vi "Send Data.vi"() -> ()   [LabVIEW 2020, in "RT_Cluster.lvclass"]
uses:
  RT_Cluster.lvclass
  Desktop/efr_12/02_Electronics/VCU/Software/Project_EFR12e09/Typedefs/RT_Cluster.ctl
  Desktop/efr_12/02_Electronics/VCU/Software/Project_EFR12e09/Typedefs/RT_Vehicle_Modes.ctl
  RT_Cluster.lvclass/RT_Cluster.ctl
  <vilib>/Platform/TimedLoop/XDataNode/timing_clust.ctl
  <vilib>/Platform/TimedLoop/XDataNode/nitl_modes.ctl
  <vilib>/Platform/TimedLoop/XDataNode/wakeup.ctl
  944b02c2-96e3-4360-906f-94be907d6afc.vi
  52bb762b-3344-4100-a38b-be0fe8b4f671.vi
  743889c7-9139-4068-ac03-3bcab9db493b.vi
  7bc09824-a4a5-4f1b-b862-42a96e625018.vi
  c340d439-48fc-4ce6-b793-888df5355522.vi
  fd4fa075-0ab3-44ce-9a90-155efef00941.vi
  f70b0d1b-d714-4ea4-9e83-26cb66d79a99.vi
  c65facf9-95a3-4195-afb2-c6ea00a184ea.vi
  <vilib>/JDP Science/JSONtext/Variant to JSON Text.vi
  <vilib>/JDP Science/JSONtext/LVClass Serializer/JSONtext LVClass Serializer.lvclass
  <vilib>/platform/TimedLoop/XDataNode/XDataNode.xnode
  <vilib>/Platform/TimedLoop/XDataNode/XDNodeRunTimeDep.lvlib
panel:
  in  "Vehicle Mode":T1
  out "<JSON> 8":string
  out "<JSON> 7":string
  out "<JSON> 6":string
  out "<JSON> 5":string
  out "<JSON> 4":string
  out "<JSON> 3":string
  out "<JSON> 2":string
  out "<JSON>":string
  out "concatenated string":string
  out "xml string":string
  out "port":refnum<k16>
  out "send structure":dbl
  out "String 6":string
  out "Numeric":dbl
  out "String 5":string
  out "String 4":string
  out "String 2":string
  in  "stop 17":bool
  in  "stop 15":bool
  in  "stop 13":bool
  in  "stop 11":bool
  in  "stop 8":bool
  in  "stop 6":bool
  in  "stop 5":bool
  in  "stop 2":bool
  in  "Timestamp":cluster{"Timestamp":timestamp}
  in  "RT_Cluster.lvclass":T2
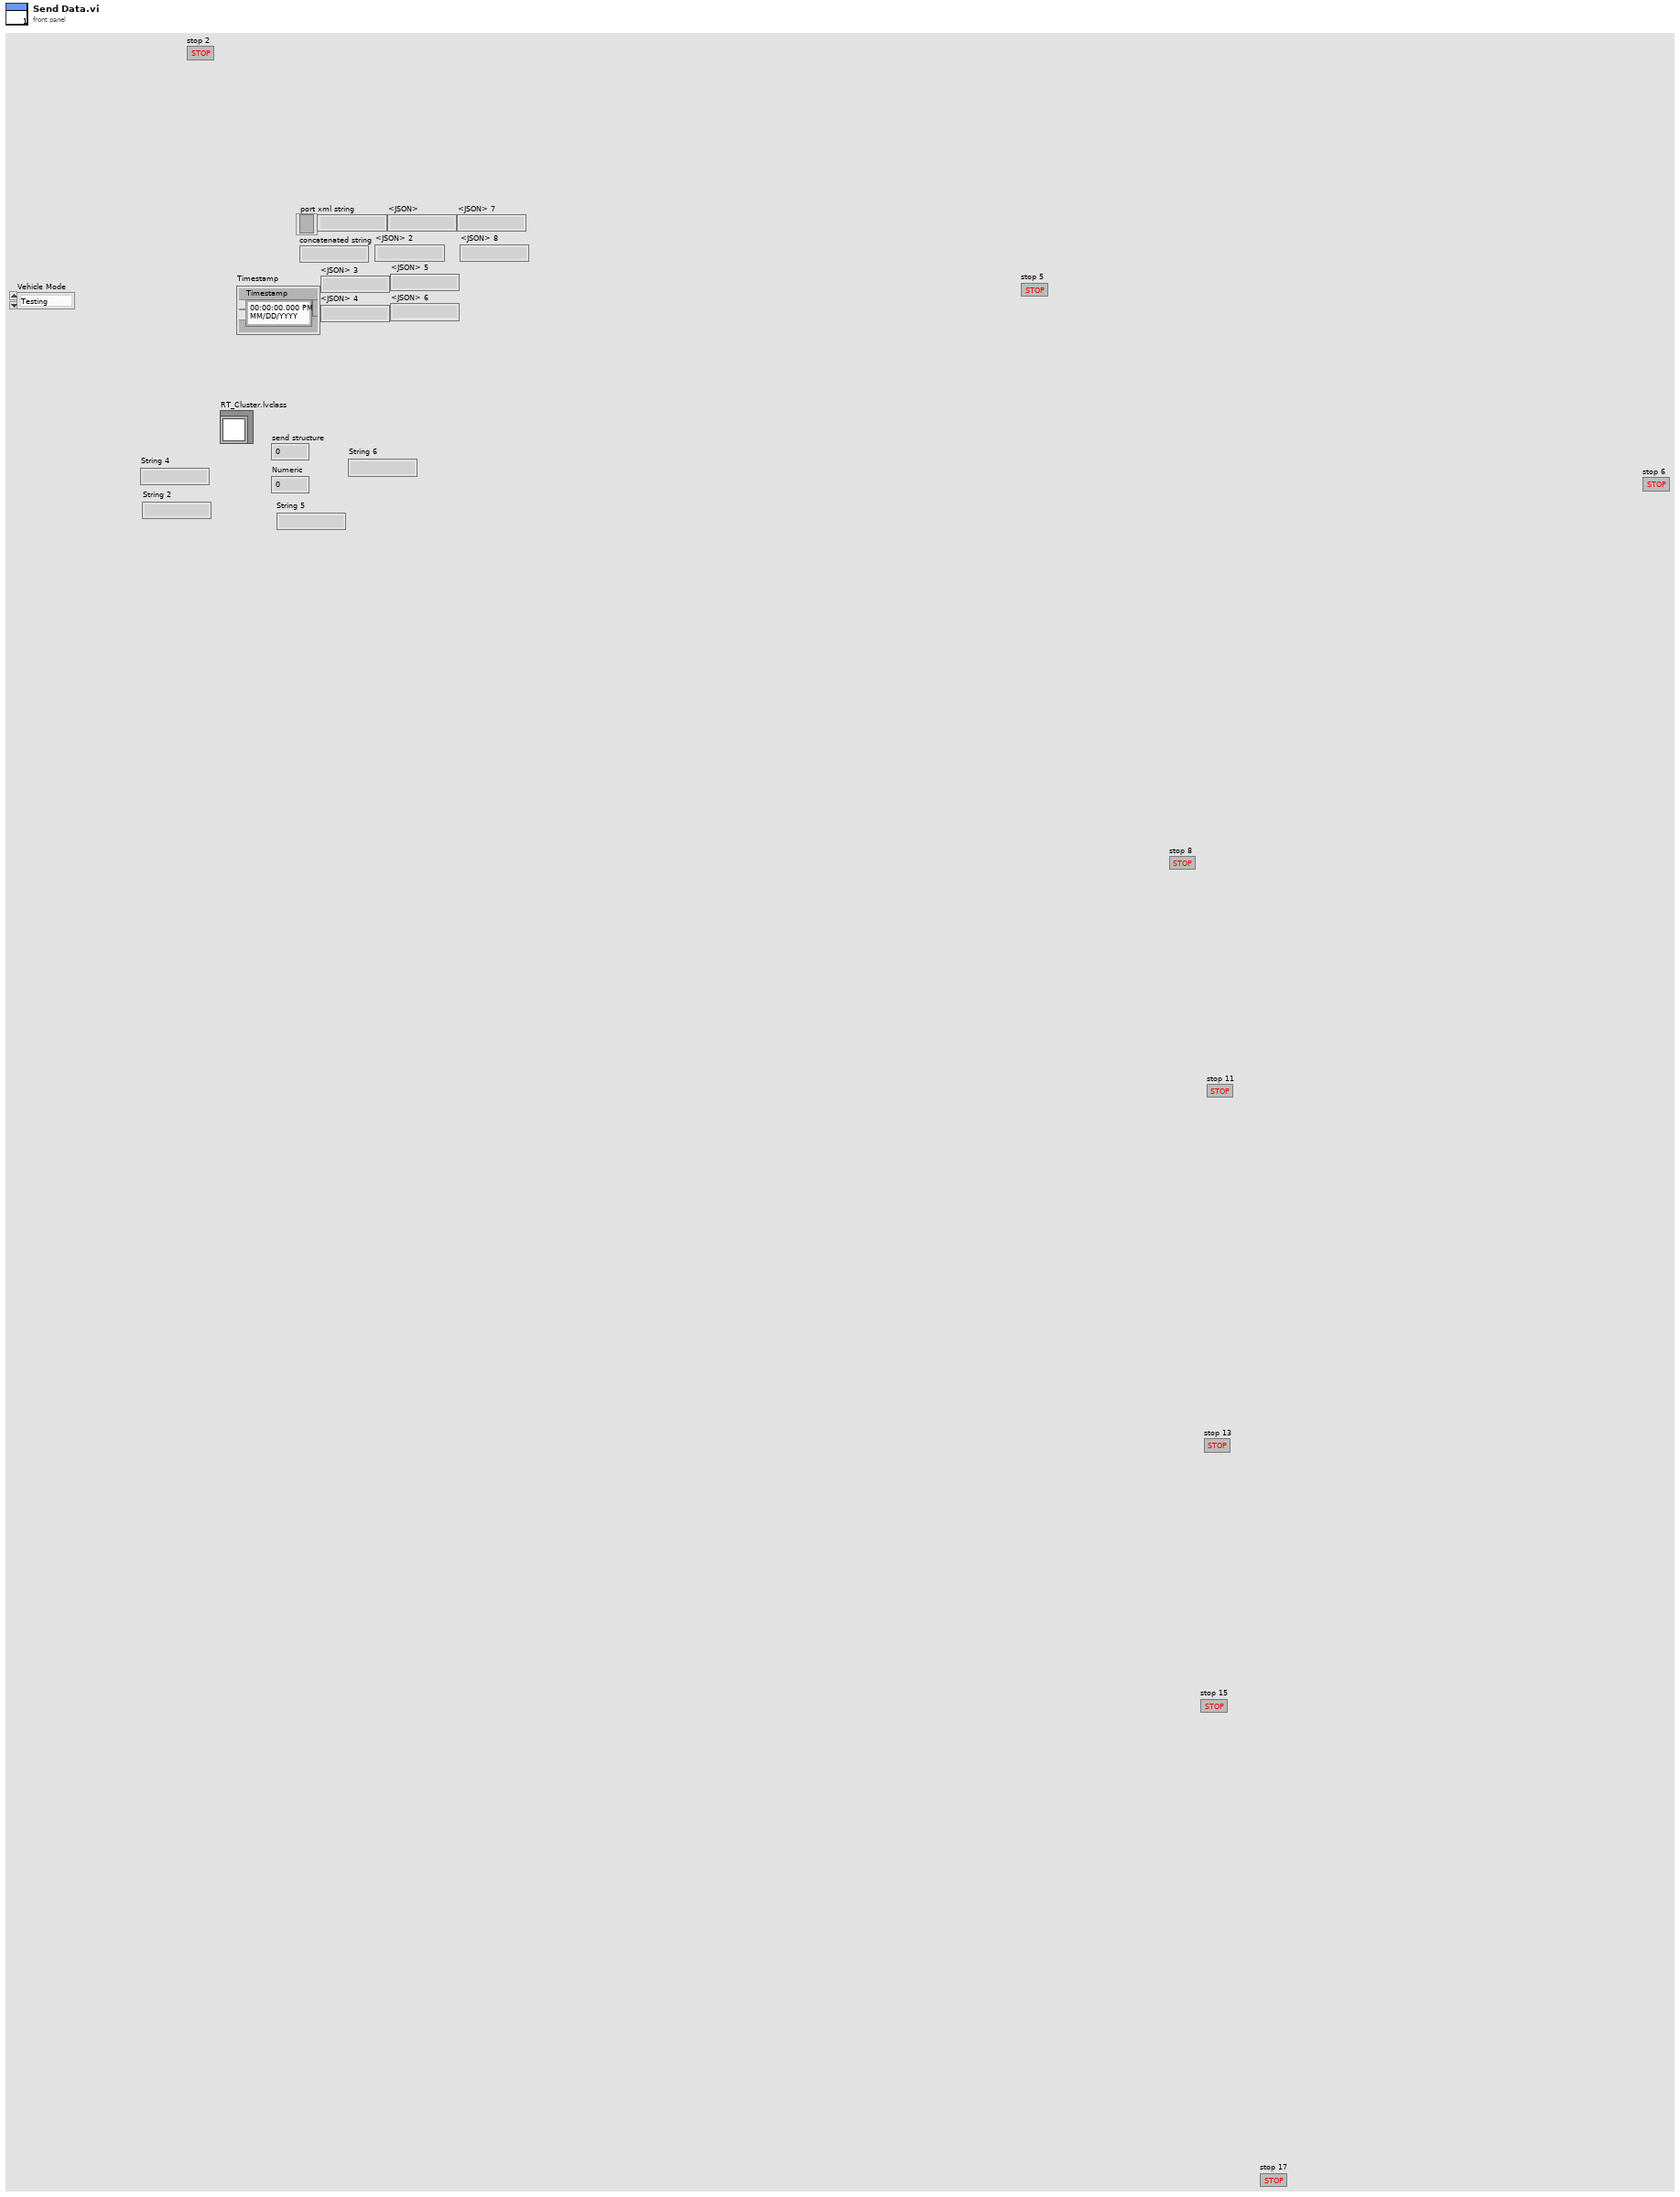
[diagram p1: front panel]
types:
  T1 = typedef "RT_Vehicle_Modes.ctl" = enum8{"Testing", "Scruti", "Acceleration", "Skidpad", "Autocross", "Endurance"}
  T2 = typedef "RT_Cluster.ctl" = refnum<class "RT_Cluster.lvclass">
  T3 = enum16{"big-endian, network order", "native, host order", "little-endian"}
  T4 = cluster{"Vehicle Mode":T1, "APPS1_min[°]":sgl, "APPS1_max[°]":sgl, "APPS2_min[°]":sgl, "APPS2_max[°]":sgl, "maxTorque+[Nm]":sgl, "maxTorque-[Nm]":sgl, "Leistungslimit[kW]":sgl, "maxRPM[1/min]":sgl, "Rekuperation":bool, "ASR":bool, "BSR":bool, "TV":bool, "DRS":bool, "Energiesparmodus":bool, "Accelslip [%/100]":sgl, "Brakeslip [%/100]":sgl, "Backupload":bool, "Config locked":bool, "InverterVR-active":bool, "InverterVL-active":bool, "InverterHR-active":bool, "InverterHL-active":bool}
  T5 = typedef "RT_AMS_States.ctl" = enum8{"Idle", "Precharging", "Drive", "reserved", "Precharge Failed", "Data Error", "Relay(s) stuck"}
  T6 = typedef "RT_IMD_States.ctl" = enum8{"IMD aus", "PWM nicht erkannt", "Normal", "Unterspannung", "Schnellstartmessung gut", "Schnellstartmessung schlecht", "Gerätefehler", "Anschlussfehler Erde"}
  T7 = typedef "FPGA_RT_Fuses.ctl" = cluster{"Fuse1[b]":bool, "Fuse2_SSB[b]":bool, "Fuse3_IMD[b]":bool, "Fuse4_Inv[b]":bool, "Fuse5_GPS[b]":bool, "Fuse6_VCU[b]":bool, "Fuse7_BSE[b]":bool, "Fuse8_DIS[b]":bool, "Fuse9_SWS[b]":bool, "Fuse10_TPMS[b]":bool, "Fuse11[b]":bool, "Fuse12[b]":bool, "Fuse1A_1_RTDS":bool, "Fuse1A_2_Brakelight":bool, "Fuse1A_3":bool, "Fuse1A_4":bool, "Fuse6A_1_Motor_Fans":bool, "Fuse6A_2_DRS":bool, "Fuse6A_3_SC":bool, "Fuse6A_4_Vectorbox":bool, "Fuse6A_5_Mot_Pumps":bool, "Fuse6A_6":bool, "Fuse12A_1_Inv_Fans_Fr":bool, "Fuse12A_2_Inv_Fans_Re":bool}
  T8 = cluster{"Analog":cluster{"APPS1[°]":sgl, "APPS2[°]":sgl, "Bremsdruck vorne [bar]":sgl, "Bremsdruck hinten [bar]":sgl, "Bremskraft[N]":sgl, "Lenkwinkel[°]":sgl, "WT_Motor_high[°C]":sgl, "WT_Motor_Low[°C]":sgl, "LT_Inv_FrR[°C]":sgl, "LT_Inv_FrL[°C]":sgl, "LT_Inv_ReR[°C]":sgl, "LT_Inv_ReL[°C]":sgl, "Ambient_Temp[°C]":sgl, "ST_FR[mm}":sgl, "ST_FL[mm]":sgl, "ST_RR[mm]":sgl, "ST_RL[mm]":sgl, "Temp_Fusebox [°C]":sgl}, "Akku/HV":cluster{"HV_Current[A]":sgl, "IC_Voltage[V]":sgl, "Charge[Ah]":sgl, "AMS-State":T5, "State SC":bool, "Akku-Voltage[V]":sgl, "SOC[%]":sgl, "CVH[V]":sgl, "CVL[V]":sgl, "CVL[V] 20s":sgl, "CVL[V] 60s":sgl, "CTH[°C]":sgl, "CTL[°C]":sgl, "State IMD":T6, "Isolationswider\nstand[kOhm]":u16}, "SC":cluster{"SC Messungen":cluster{"SC after Motors Rear [V]":sgl, "SC after Motors Front [V]":sgl, "SC after BOTS [V]":sgl, "SC after Akku [V]":sgl, "SC Voltage AMS 1":sgl, "SC Voltage AMS 2":sgl}, "SC Errors":cluster{"SC Motors Front":bool, "SC Motors Rear":bool, "SC BOTS":bool, "SC Akku":bool}}, "Fuses":T7, "Buttons/Knobs":cluster{"TunKnob 1[%]":sgl, "TunKnob 2[%]":sgl, "Start-Button":bool, "HV-Button":bool, "Reku-Button":bool, "Lenkrad 1":bool, "Lenkrad 2":bool, "Lenkrad 3":bool, "Lenkrad 4":bool, "Lenkrad 5":bool, "Lenkrad 6":bool}, "GPS/9-axis Front":cluster{"V_GPS[km/h]":sgl, "Course_GPS[°]":sgl, "Latitude[°]":dbl, "Longitude[°]":dbl, "HDOP":u8, "Quality of Fix":u8, "Satellites":u8, "Odometer[km]":sgl, "ACC_X_Fr[m/s²]":sgl, "ACC_Y_Fr[m/s²] ":sgl, "ACC_Z_Fr[m/s²]":sgl, "ROT_X_Fr[°/s]":sgl, "ROT_Y_Fr[°/s]":sgl, "ROT_Z_Fr[°/s]":sgl, "MAG_X_Fr[b]":sgl, "MAG_Y_Fr[b]":sgl, "MAG_Z_Fr[b]":sgl}, "GPS/9-axis Rear":cluster{"V_GPS[km/h]":sgl, "Course_GPS[°]":sgl, "Latitude[°]":dbl, "Longitude[°]":dbl, "HDOP":u16, "Quality of Fix":u16, "Satellites":u16, "Odometer[km]":sgl, "ACC_X_Re[m/s²]":sgl, "ACC_Y_Re[m/s²] ":sgl, "ACC_Z_Re[m/s²]":sgl, "ROT_X_Re[°/s]":sgl, "ROT_Y_Re[°/s]":sgl, "ROT_Z_Re[°/s]":sgl, "MAG_X_Re[b]":sgl, "MAG_Y_Re[b]":sgl, "MAG_Z_Re[b]":sgl}, "Fusebox Currents":cluster{"1A_1":sgl, "1A_ 2":sgl, "1A_3":sgl, "1A_4":sgl, "6A_1":sgl, "6A_2":sgl, "6A_3":sgl, "6A_4":sgl, "6A_5":sgl, "6A_6":sgl, "12A_1":sgl, "12A_2":sgl}, "Kistler":cluster{"Timestamp [4ms] ":u16, "IVI [10^-2 m/s]":u16, "Weg [m]":sgl, "V_lon [m/s]":sgl, "V_lat [m/s]":sgl, "Winkel [°]":sgl, "SerienNr":u32, "SensorNr":u8, "Temp [°C]":i8, "LED Strom [0,01A]":u8, "Statusbyte1":u8, "Statusbyte2":u8}, "Datalogger":cluster{"Status":u8, "Voltage[V]":sgl, "Current[A]":sgl, "Power[kW]":sgl, "Message\nCounter":sgl}}
  T9 = typedef "RT_Inverter.ctl" = cluster{"AMK_Control[b]":T10, "Drehzahlsollwert[1/min]":sgl, "Momentsollwert[Nm]":sgl, "System bereit":bool, "Warnung":bool, "Fehler":bool, "Derating":bool, "Spiegel HV":bool, "Quit HV":bool, "Spiegel Regelerfeigabe":bool, "Quit Reglerfreigabe":bool, "Drehzahlistwert[U/min]":sgl, "Momentistwert[Nm]":sgl, "Diagnosenummer":u16, "Motortemp[°C]":sgl, "Kühlplattentemp[°C]":sgl, "IGBTtemp[°C]":sgl, "I_q[A]":sgl, "I_d[A]":sgl, "Wirkleistung [kW]":sgl, "Blindleistung [kvar]":sgl, "Fehlerzusatznr. 1":u8, "Fehlerzusatznr. 2":u8, "Fehlerzusatznr. 3":u8}
  T10 = typedef "RT_AMK_Control.ctl" = enum8{"Fehler zurücksetzen", "HV-Freigabe", "HV+Antriebsfreigabe", "HV+Antriebs+Reglerfreigabe"}
  T11 = typedef "RT_Errors.ctl" = cluster{"Timeout CAN":T12, "Wert":cluster{"Pedale implausibel":bool, "APPS implausibel":bool, "APPS1":bool, "APPS2":bool, "Bremsdruck_vorne":bool, "Bremsdruck_hinten":bool, "Bremskraftsensor":bool, "Lenkwinkel":bool, "ACC_X":bool, "ACC_Y":bool, "ROT_Z":bool, "V_GPS":bool, "Invertertemp_FrR":bool, "Invertertemp_FrL":bool, "Invertertemp_ReR":bool, "Invertertemp_ReL":bool}, "Latching":cluster{"Pedale implausibel":bool, "APPS implausibel":bool, "APPS1":bool, "APPS2":bool}}
  T12 = typedef "FPGA_To_RT_CANErrors.ctl" = cluster{"SSB Front":bool, "BSE":bool, "SSB Rear":bool, "GPS Front":bool, "9-Achs_ACC Front":bool, "9-Achs_ROT Front":bool, "9-Achs_MAG Front":bool, "GPS Rear":bool, "9-Achs_ACC Rear":bool, "9-Achs_ROT Rear":bool, "9-Achs_MAG Rear":bool, "AMS":bool, "Energymeter":bool, "PDU":bool, "DIS":bool, "DIS_Param":bool, "Inverter FR":bool, "Inverter FL":bool, "Inverter RR":bool, "Inverter RL":bool}
  T13 = typedef "RT_Maths.ctl" = cluster{"General":cluster{"desiredTorque[Nm]":sgl, "Gaspedal[%/100]":sgl, "Rekupedal[%/100]":sgl, "Implausibilität\nAPPS[%]":sgl, "Bremsbal[Fr/Total]":sgl, "Accelbal[Fr/Total]":sgl, "allowedPower[kW]":sgl, "actualPower[kW]":sgl, "Energiesparmodus":bool, "Odometer":sgl, "Wirkungsgrad[%/100]":sgl, "T_Control[us]":sgl}, "TV/KF":cluster{"KF_Velocity[km/h]":sgl, "KF_ACC_X[m/s²]":sgl, "KF_slip_ist_FR[%/100]":sgl, "KF_slip_ist_FL[%/100]":sgl, "KF_slip_ist_RR[%/100]":sgl, "KF_slip_ist_RL[%/100]":sgl, "slip_soll_Fr[%/100]":sgl, "slip_soll_Re[%/100]":sgl, "TV_Regler[Giermoment]":sgl, "TV_Lenk[Giermoment]":sgl, "SOC-Soll[%]":sgl, "SOC-Ist[%]":sgl, "MomentSollVR[Nm]":sgl, "MomentSollVL[Nm]":sgl, "MomentSollHR[Nm]":sgl, "MomentSollHL[Nm]":sgl, "Reglerausgang":sgl}, "Energy Control":cluster{"allowedPower[kW]":sgl, "Rundenanzahl":sgl, "SOC-Soll[%]":sgl, "SOC-Ist[%]":sgl, "Rundenlänge[m]":sgl, "Reglerausgang":sgl, "Toleranz Rundenlänge [%/100]":sgl, "Strecke":T14, "Start-SOC[%]":sgl, "Ziel-SOC[%]":sgl, "Energie Akku[kWh]":sgl, "Maximalleistung[kW]":sgl, "Start-Leistungsgrenze":sgl}}
  T14 = typedef "RT_Tracks.ctl" = enum16{"Freital", "Barcelona", "Hockenheim", "Spielberg", "Assen"}
  T15 = typedef "RT_Vehicle_States.ctl" = enum8{"Idle", "Drive", "Error"}
  T16 = cluster{"Switches":cluster{"\n1A 1 RTDS":bool, "1A 2 Brakelight":bool, "1A 3":bool, "1A 4":bool, "6A 1 Motor Fans":bool, "6A 2 DRS":bool, "6A 3 SC":bool, "6A 4 Vectorbox":bool, "6A 5 Motor Pump":bool, "6A 6":bool, "12A 1 Inv Fans Fr":bool, "12A 2 Inv Fans Re":bool}, "Vehicle State":T15, "DRS Position[%/100]":sgl, "Fan Motor[%/100]":sgl, "Fan Akku[%/100]":sgl, "HV Freigabe ":bool, "IC Voltage OK":bool}
  T17 = cluster{"Input Error Code":i32, "Output Error Code":i32, "Transmit Error Counter":u8, " Error Counter":u32}
  T18 = typedef "XDNodeRunTimeDep.lvlib/timing_clust.ctl" = cluster{"Expected End [f-1]":u64, "Actual End [f-1]":u64, "Finished Late? [f-1]":bool, "Expected End [i-1]":u64, "Actual End [i-1]":u64, "Finished Late? [i-1]":bool, "Expected Start [i]":u64, "Actual Start [i]":u64, "Expected Start [f]":u64, "Actual Start [f]":u64, "Source Name":string, "Structure Name":string, "Period":i64, "Deadline":i64, "Offset":i64, "Start":i64, "Priority":i32, "Timeout":i32, "Mode":T19, "Wakeup Reason":T20, "Error":errorcluster, "Source Type":string, "Secondary Source Type":string, "Global End Time":u64, "Global Start Time":u64, "Frame Duration":u64, "Iteration Duration":u64, "Assigned CPU":i32, "I/O Scan Engine Mode":u32}
  T19 = typedef "XDNodeRunTimeDep.lvlib/nitl_modes.ctl" = enum32{"No Change", "Process missed periods, maintain original phase", "Discard missed periods, maintain original phase", "Process missed periods, ignore original phase", "Discard missed periods, ignore original phase"}
  T20 = typedef "XDNodeRunTimeDep.lvlib/wakeup.ctl" = enum32{"Normal", "Aborted", "Asynchronous wakeup", "Timing source error", "Timed loop error", "Timeout"}
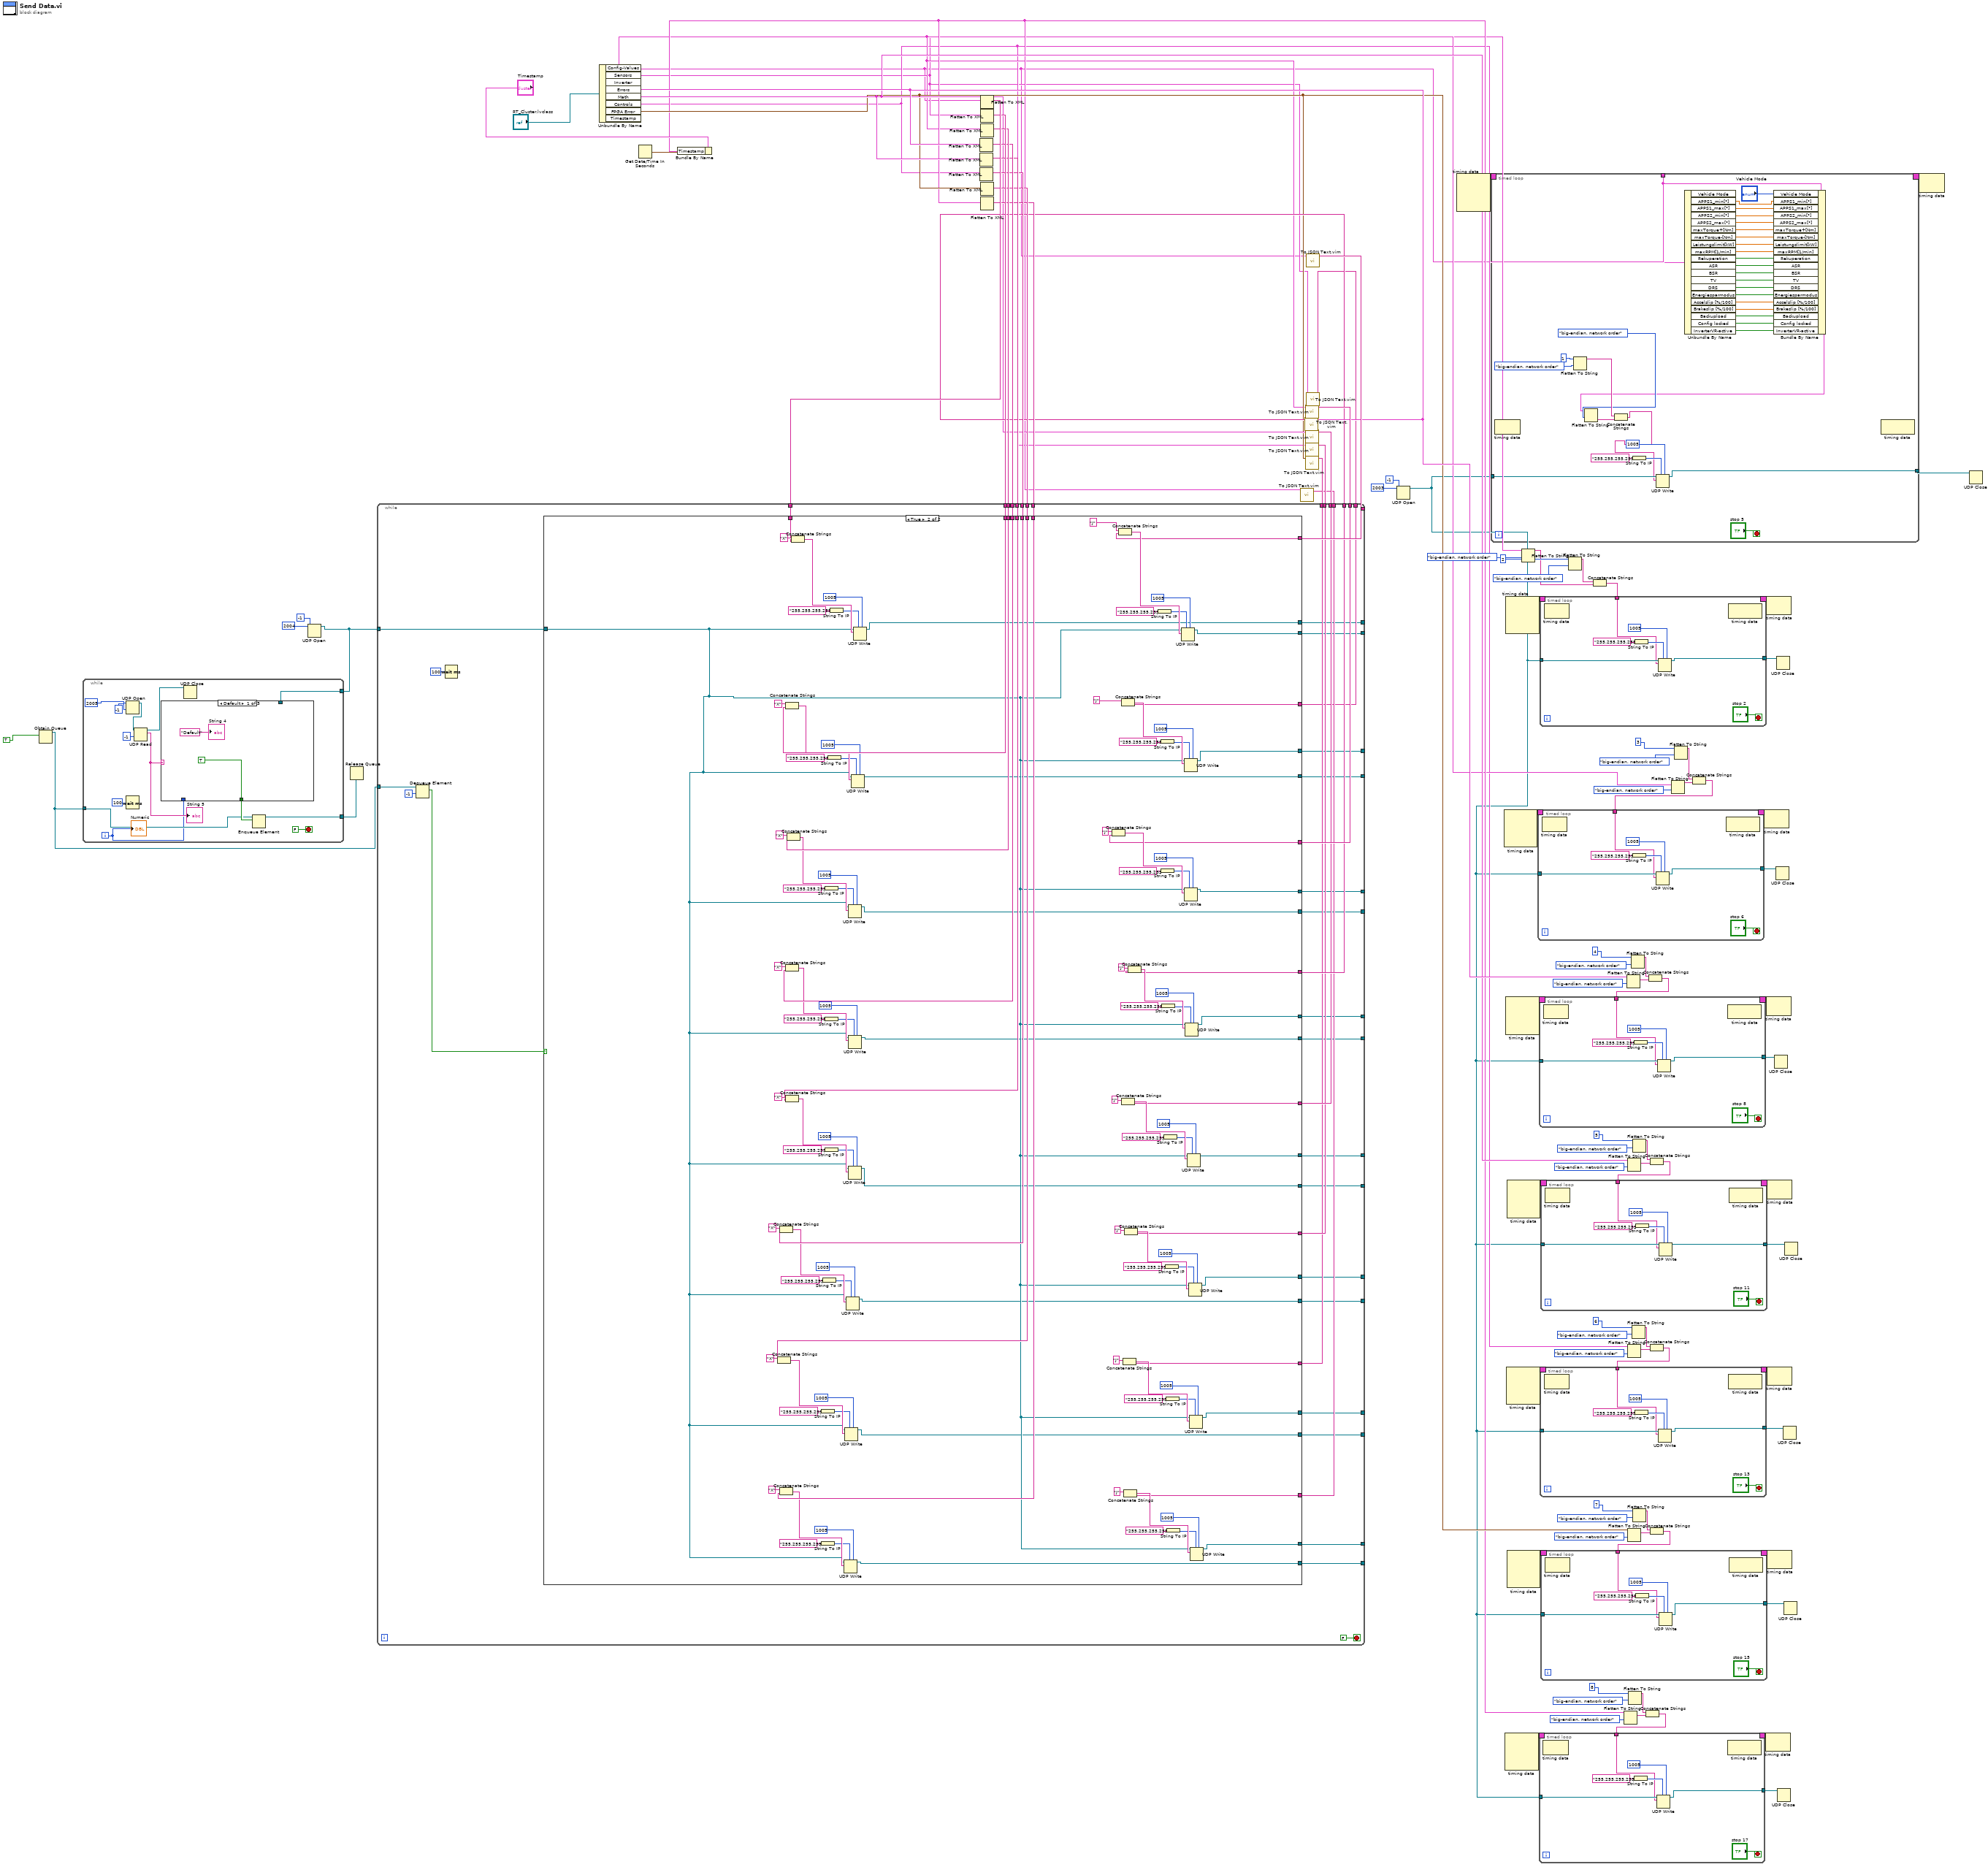
[diagram p0: block diagram]
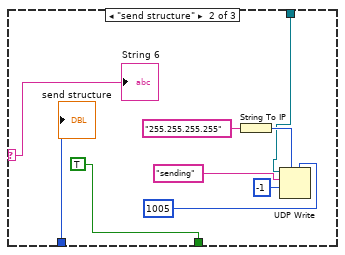
[diagram p2: hidden frame]
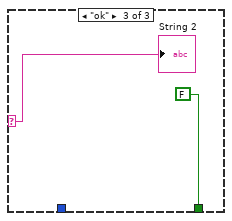
[diagram p3: hidden frame]
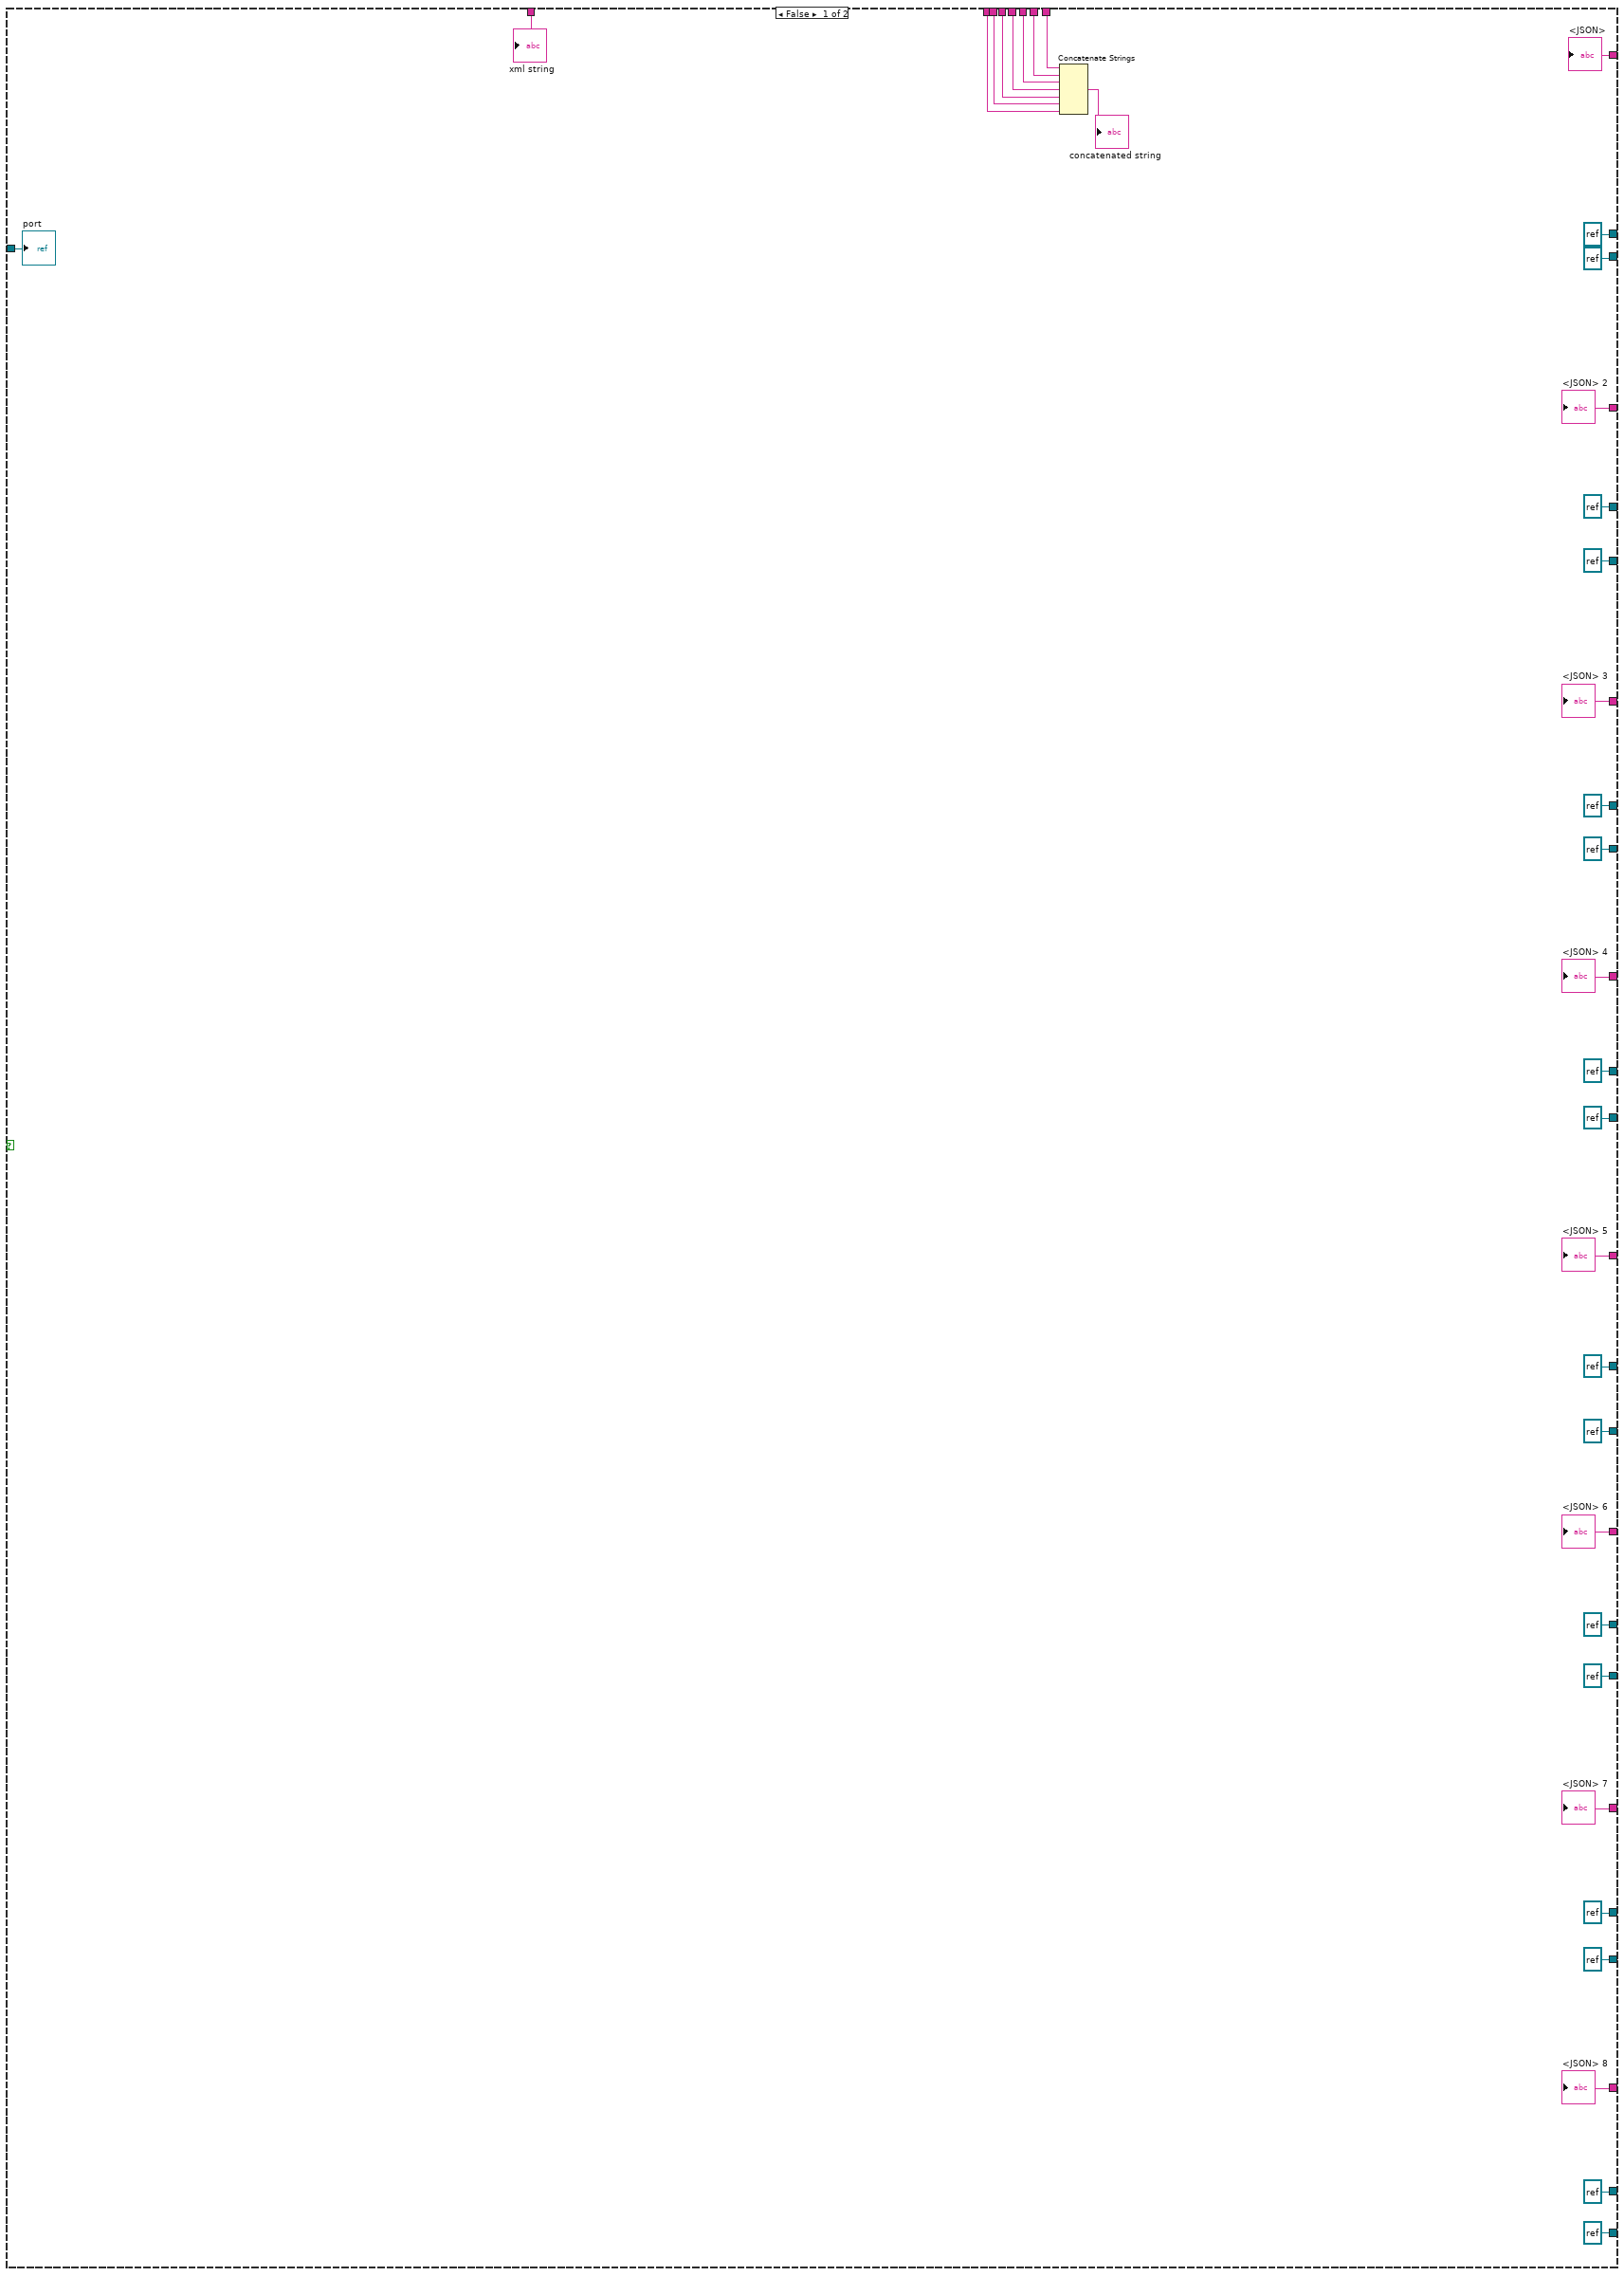
[diagram p4: hidden frame]
diagram:
  n1 = Obtain Queue(element data type=TRUE) -> (queue out=w2:refnum<queue>)  [unwired: 4 in, 2 out]
  n2 = UDP Open(9:-1 ("timeout ms (25000)"), 11:u16 2004 ("port")) -> (port=w5:refnum<k16>)  [unwired: 3 in, 2 out]
  n3 = while {
    tunnel: w5 -> [w115]
    tunnel: w2 -> [w109]
    tunnel: [w111] -> w3
    i -> [w103]
    stop <- FALSE stop-if-true
    n4 = UDP Open(9:-1 ("timeout ms (25000)"), 11:u16 2005 ("port")) -> (port=w104:refnum<k16>)  [unwired: 3 in, 2 out]
    n5 = Wait (ms)(milliseconds to wait=u32 100) -> ()  [unwired: 1 out]
    n6 = UDP Read(connection ID=w104, timeout ms (25000)=-1) -> (data out=w108:string, 3:w107:refnum<k16>)  [unwired: 2 in, 3 out]
    "String 5" <- w108
    n7 = case shown="Default" w108 {
      selector: w108 -> [_ w119 w127]
      tunnel: [TRUE TRUE FALSE] -> w110
      tunnel: w115 -> [_ w120 _]
      tunnel: w103 -> [_ w118 _]
      frame Default {
        "String 4" <- "Default" ("String 2")
      }
      frame "send structure" {
        n8 = String To IP(1:"255.255.255.255" ("name")) -> (0:w126:u32)
        n9 = UDP Write(address=w126, port or service name=u16 1005, connection ID=w120, data in="sending", 9:-1 ("timeout ms (25000)")) -> ()  [unwired: 1 in, 2 out]
        "String 6" <- w119
        "send structure" <- w118
      }
      frame "ok" {
        "String 2" <- w127
      }
    }
    n10 = UDP Close(connection ID=w107) -> ()  [unwired: 1 in, 2 out]
    n11 = Enqueue Element(queue=w109, element=w110) -> (queue out=w111:refnum<queue>)  [unwired: 2 in, 2 out]
    "Numeric" <- w103
  }
  n12 = Release Queue(queue=w3) -> ()  [unwired: 2 in, 3 out]
  n13 = Unbundle By Name("RT_Cluster.lvclass") -> ("Config-Values"=w1:T4, "Sensors"=w18:T8, "Inverter"=w21:cluster{"VR":T9, "VL":T9, "HR":T9, "HL":T9}, "Errors"=w57:T11, "Math"=w48:T13, "Controls"=w19:T16, "FPGA Error"=w33:T17)  [unwired: 1 out]
  n14 = Get Date/Time In Seconds() -> (seconds since 1Jan1904=w31:timestamp)
  n15 = Bundle By Name(cluster="Timestamp", "Timestamp"=w31) -> (w23:cluster{"Timestamp":timestamp})
  n16 = Flatten To XML(6:w57) -> (2:w75:string)
  n17 = Flatten To XML(6:w48) -> (2:w74:string)
  n18 = Flatten To XML(6:w19) -> (2:w73:string)
  n19 = Flatten To XML(6:w21) -> (2:w76:string)
  n20 = Flatten To XML(6:w33) -> (2:w72:string)
  n21 = Flatten To XML(6:w1) -> (2:w78:string)
  n22 = Flatten To XML(6:w18) -> (2:w77:string)
  n23 = Flatten To XML(6:w23) -> (2:w71:string)
  n24 = call "To JSON Text.vim"("Anything"=w23) -> ("<JSON>"=w30:string)  [unwired: 9 in, 1 out]
  n25 = call "To JSON Text.vim"("Anything"=w57) -> ("<JSON>"=w56:string)  [unwired: 9 in, 1 out]
  n26 = call "To JSON Text.vim"("Anything"=w21) -> ("<JSON>"=w64:string)  [unwired: 9 in, 1 out]
  n27 = call "To JSON Text.vim"("Anything"=w48) -> ("<JSON>"=w55:string)  [unwired: 9 in, 1 out]
  n28 = call "To JSON Text.vim"("Anything"=w19) -> ("<JSON>"=w47:string)  [unwired: 9 in, 1 out]
  n29 = call "To JSON Text.vim"("Anything"=w33) -> ("<JSON>"=w40:string)  [unwired: 9 in, 1 out]
  n30 = call "To JSON Text.vim"("Anything"=w1) -> ("<JSON>"=w79:string)  [unwired: 9 in, 1 out]
  n31 = call "To JSON Text.vim"("Anything"=w18) -> ("<JSON>"=w20:string)  [unwired: 9 in, 1 out]
  n32 = while {
    tunnel: w79 -> [w166]
    tunnel: w78 -> [w165]
    tunnel: w77 -> [w164]
    tunnel: w76 -> [w163]
    tunnel: w75 -> [w162]
    tunnel: w74 -> [w161]
    tunnel: w73 -> [w160]
    tunnel: w72 -> [w159]
    tunnel: w71 -> [w158]
    tunnel: w64 -> [w157]
    tunnel: w56 -> [w156]
    tunnel: w55 -> [w155]
    tunnel: w47 -> [w154]
    tunnel: w40 -> [w153]
    tunnel: w30 -> [w152]
    tunnel: w20 -> [w151]
    tunnel: w5 -> [w150]
    tunnel: [w149] -> _
    tunnel: [w148] -> _
    tunnel: [w147] -> _
    tunnel: [w146] -> _
    tunnel: [w145] -> _
    tunnel: [w144] -> _
    tunnel: [w143] -> _
    tunnel: [w142] -> _
    tunnel: [w141] -> _
    tunnel: [w140] -> _
    tunnel: [w139] -> _
    tunnel: [w138] -> _
    tunnel: [w137] -> _
    tunnel: [w136] -> _
    tunnel: [w135] -> _
    tunnel: [w134] -> _
    tunnel: w2 -> [w132]
    stop <- FALSE stop-if-true
    n33 = Dequeue Element(queue=w132, timeout in ms (-1)=-1) -> (element=w130:bool)  [unwired: 1 in, 3 out]
    n34 = Wait (ms)(milliseconds to wait=u32 100) -> ()  [unwired: 1 out]
    n35 = case shown="True" w130 {
      tunnel: w166 -> [w190 w312]
      tunnel: w165 -> [w199 w201]
      tunnel: w164 -> [w192 w299]
      tunnel: w163 -> [w193 w297]
      tunnel: w162 -> [w194 w295]
      tunnel: w161 -> [w195 w293]
      tunnel: w160 -> [w196 w291]
      tunnel: w159 -> [w197 w289]
      tunnel: w158 -> [w198 w287]
      tunnel: w157 -> [w184 w283]
      tunnel: w156 -> [w181 w280]
      tunnel: w155 -> [w178 w277]
      tunnel: w154 -> [w175 w274]
      tunnel: w153 -> [w172 w271]
      tunnel: w152 -> [w169 w268]
      tunnel: w151 -> [w187 w267]
      tunnel: w150 -> [w200 w218]
      tunnel: [refnum<k16> refnum ("connection ID out") w217] -> w149
      tunnel: [refnum<k16> refnum ("connection ID out") w216] -> w148
      tunnel: [refnum<k16> refnum ("connection ID out") w215] -> w147
      tunnel: [refnum<k16> refnum ("connection ID out") w214] -> w146
      tunnel: [refnum<k16> refnum ("connection ID out") w213] -> w145
      tunnel: [refnum<k16> refnum ("connection ID out") w212] -> w144
      tunnel: [refnum<k16> refnum ("connection ID out") w211] -> w143
      tunnel: [refnum<k16> refnum ("connection ID out") w210] -> w142
      tunnel: [refnum<k16> refnum ("connection ID out") w209] -> w141
      tunnel: [refnum<k16> refnum ("connection ID out") w208] -> w140
      tunnel: [refnum<k16> refnum ("connection ID out") w207] -> w139
      tunnel: [refnum<k16> refnum ("connection ID out") w206] -> w138
      tunnel: [refnum<k16> refnum ("connection ID out") w205] -> w137
      tunnel: [refnum<k16> refnum ("connection ID out") w204] -> w136
      tunnel: [refnum<k16> refnum ("connection ID out") w203] -> w135
      tunnel: [refnum<k16> refnum ("connection ID out") w202] -> w134
      frame False {
        n36 = Concatenate Strings(w198, w197, w196, w195, w194, w193, w192) -> (→"concatenated string":string)
        "port" <- w200
        "xml string" <- w199
        "<JSON>" <- w190
        "<JSON> 2" <- w187
        "<JSON> 3" <- w184
        "<JSON> 4" <- w181
        "<JSON> 5" <- w178
        "<JSON> 6" <- w175
        "<JSON> 7" <- w172
        "<JSON> 8" <- w169
      }
      frame True {
        n37 = Concatenate Strings("X" ("string"), w289) -> (w288:string)
        n38 = Concatenate Strings("X" ("string"), w287) -> (w286:string)
        n39 = Concatenate Strings("X" ("string"), w291) -> (w290:string)
        n40 = Concatenate Strings("X" ("string"), w295) -> (w294:string)
        n41 = Concatenate Strings("X" ("string"), w299) -> (w298:string)
        n42 = Concatenate Strings("X" ("string"), w293) -> (w292:string)
        n43 = Concatenate Strings("X" ("string"), w297) -> (w296:string)
        n44 = Concatenate Strings("X" ("string"), w201) -> (w300:string)
        n45 = String To IP(1:"255.255.255.255" ("name")) -> (0:w245:u32)
        n46 = String To IP(1:"255.255.255.255" ("name")) -> (0:w248:u32)
        n47 = String To IP(1:"255.255.255.255" ("name")) -> (0:w251:u32)
        n48 = String To IP(1:"255.255.255.255" ("name")) -> (0:w260:u32)
        n49 = String To IP(1:"255.255.255.255" ("name")) -> (0:w254:u32)
        n50 = String To IP(1:"255.255.255.255" ("name")) -> (0:w257:u32)
        n51 = String To IP(1:"255.255.255.255" ("name")) -> (0:w263:u32)
        n52 = String To IP(1:"255.255.255.255" ("name")) -> (0:w266:u32)
        n53 = UDP Write(address=w245, port or service name=u16 1005, connection ID=w218, data in=w286) -> (3:w202:refnum<k16>)  [unwired: 2 in, 1 out]
        n54 = UDP Write(address=w248, port or service name=u16 1005, connection ID=w218, data in=w288) -> (3:w204:refnum<k16>)  [unwired: 2 in, 1 out]
        n55 = UDP Write(address=w251, port or service name=u16 1005, connection ID=w218, data in=w290) -> (3:w206:refnum<k16>)  [unwired: 2 in, 1 out]
        n56 = UDP Write(address=w260, port or service name=u16 1005, connection ID=w218, data in=w296) -> (3:w212:refnum<k16>)  [unwired: 2 in, 1 out]
        n57 = UDP Write(address=w254, port or service name=u16 1005, connection ID=w218, data in=w292) -> (3:w208:refnum<k16>)  [unwired: 2 in, 1 out]
        n58 = UDP Write(address=w257, port or service name=u16 1005, connection ID=w218, data in=w294) -> (3:w210:refnum<k16>)  [unwired: 2 in, 1 out]
        n59 = UDP Write(address=w263, port or service name=u16 1005, connection ID=w218, data in=w298) -> (3:w214:refnum<k16>)  [unwired: 2 in, 1 out]
        n60 = UDP Write(address=w266, port or service name=u16 1005, connection ID=w218, data in=w300) -> (3:w217:refnum<k16>)  [unwired: 2 in, 1 out]
        n61 = Concatenate Strings("J" ("string"), w283) -> (w285:string)
        n62 = Concatenate Strings("J" ("string"), w312) -> (w313:string)
        n63 = Concatenate Strings("J" ("string"), w267) -> (w310:string)
        n64 = Concatenate Strings("J" ("string"), w277) -> (w279:string)
        n65 = Concatenate Strings("J" ("string"), w271) -> (w273:string)
        n66 = Concatenate Strings("J" ("string"), w268) -> (w270:string)
        n67 = Concatenate Strings("J" ("string"), w274) -> (w276:string)
        n68 = Concatenate Strings("J" ("string"), w280) -> (w282:string)
        n69 = String To IP(1:"255.255.255.255" ("name")) -> (0:w221:u32)
        n70 = String To IP(1:"255.255.255.255" ("name")) -> (0:w224:u32)
        n71 = String To IP(1:"255.255.255.255" ("name")) -> (0:w227:u32)
        n72 = String To IP(1:"255.255.255.255" ("name")) -> (0:w230:u32)
        n73 = String To IP(1:"255.255.255.255" ("name")) -> (0:w233:u32)
        n74 = String To IP(1:"255.255.255.255" ("name")) -> (0:w236:u32)
        n75 = String To IP(1:"255.255.255.255" ("name")) -> (0:w239:u32)
        n76 = String To IP(1:"255.255.255.255" ("name")) -> (0:w242:u32)
        n77 = UDP Write(address=w221, port or service name=u16 1005, connection ID=w218, data in=w313) -> (3:w216:refnum<k16>)  [unwired: 2 in, 1 out]
        n78 = UDP Write(address=w224, port or service name=u16 1005, connection ID=w218, data in=w310) -> (3:w215:refnum<k16>)  [unwired: 2 in, 1 out]
        n79 = UDP Write(address=w227, port or service name=u16 1005, connection ID=w218, data in=w285) -> (3:w213:refnum<k16>)  [unwired: 2 in, 1 out]
        n80 = UDP Write(address=w230, port or service name=u16 1005, connection ID=w218, data in=w282) -> (3:w211:refnum<k16>)  [unwired: 2 in, 1 out]
        n81 = UDP Write(address=w233, port or service name=u16 1005, connection ID=w218, data in=w279) -> (3:w209:refnum<k16>)  [unwired: 2 in, 1 out]
        n82 = UDP Write(address=w236, port or service name=u16 1005, connection ID=w218, data in=w276) -> (3:w207:refnum<k16>)  [unwired: 2 in, 1 out]
        n83 = UDP Write(address=w239, port or service name=u16 1005, connection ID=w218, data in=w273) -> (3:w205:refnum<k16>)  [unwired: 2 in, 1 out]
        n84 = UDP Write(address=w242, port or service name=u16 1005, connection ID=w218, data in=w270) -> (3:w203:refnum<k16>)  [unwired: 2 in, 1 out]
      }
    }
  }
  n85 = UDP Open(9:-1 ("timeout ms (25000)"), 11:u16 2003 ("port")) -> (port=w6:refnum<k16>)  [unwired: 3 in, 2 out]
  n86 = node-c288() -> (w100:T18)  [unwired: 4 in]
  n87 = timed-loop {
    tunnel: w6 -> [w347]
    timing: w100 -> [_]
    timing-out: [_] -> w99
    tunnel: [w342] -> w9
    tunnel: w1 -> [w335]
    stop <- "stop 5" stop-if-true
    n88 = node-c288() -> ()  [unwired: 1 in, 1 out]
    n89 = Flatten To String(anything=1 ("number"), byte order (0:big-endian, network order)=T3."big-endian, network order") -> (data string=w338:string)  [unwired: 2 in, 2 out]
    n90 = String To IP(1:"255.255.255.255" ("name")) -> (0:w346:u32)
    n91 = Unbundle By Name(w335) -> ("APPS1_min[°]"=w333:sgl, "APPS1_max[°]"=w332:sgl, "APPS2_min[°]"=w331:sgl, "APPS2_max[°]"=w330:sgl, "maxTorque+[Nm]"=w329:sgl, "maxTorque-[Nm]"=w328:sgl, "Leistungslimit[kW]"=w327:sgl, "maxRPM[1/min]"=w326:sgl, "Rekuperation"=w325:bool, "ASR"=w324:bool, "BSR"=w323:bool, "TV"=w322:bool, "DRS"=w321:bool, "Energiesparmodus"=w320:bool, "Accelslip [%/100]"=w319:sgl, "Brakeslip [%/100]"=w318:sgl, "Backupload"=w317:bool, "Config locked"=w316:bool, "InverterVR-active"=w315:bool)  [unwired: 1 out]
    n92 = Bundle By Name(cluster=w335, "Vehicle Mode"="Vehicle Mode", "APPS1_min[°]"=w333, "APPS1_max[°]"=w332, "APPS2_min[°]"=w331, "APPS2_max[°]"=w330, "maxTorque+[Nm]"=w329, "maxTorque-[Nm]"=w328, "Leistungslimit[kW]"=w327, "maxRPM[1/min]"=w326, "Rekuperation"=w325, "ASR"=w324, "BSR"=w323, "TV"=w322, "DRS"=w321, "Energiesparmodus"=w320, "Accelslip [%/100]"=w319, "Brakeslip [%/100]"=w318, "Backupload"=w317, "Config locked"=w316, "InverterVR-active"=w315) -> (w314:T4)
    n93 = Flatten To String(anything=w314, byte order (0:big-endian, network order)=T3."big-endian, network order") -> (data string=w341:string)  [unwired: 2 in, 2 out]
    n94 = Concatenate Strings(w338, w341) -> (w337:string)
    n95 = UDP Write(address=w346, port or service name=u16 1005, connection ID=w347, data in=w337) -> (3:w342:refnum<k16>)  [unwired: 2 in, 1 out]
    n96 = node-c288() -> ()  [unwired: 1 in, 1 out]
  }
  n97 = node-c288() -> (w98:T18)  [unwired: 4 in]
  n98 = node-c288() -> (w88:T18)  [unwired: 4 in]
  n99 = node-c288() -> (w96:T18)  [unwired: 4 in]
  n100 = node-c288() -> (w102:T18)  [unwired: 4 in]
  n101 = node-c288() -> (w92:T18)  [unwired: 4 in]
  n102 = node-c288() -> (w94:T18)  [unwired: 4 in]
  n103 = node-c288() -> (w90:T18)  [unwired: 4 in]
  n104 = Flatten To String(anything=w18, byte order (0:big-endian, network order)=T3."big-endian, network order") -> (data string=w81:string)  [unwired: 2 in, 2 out]
  n105 = Flatten To String(anything=2 ("number"), byte order (0:big-endian, network order)=T3."big-endian, network order") -> (data string=w85:string)  [unwired: 2 in, 2 out]
  n106 = Concatenate Strings(w85, w81) -> (w86:string)
  n107 = timed-loop {
    tunnel: w6 -> [w356]
    tunnel: w86 -> [w352]
    timing: w102 -> [_]
    timing-out: [_] -> w101
    tunnel: [w350] -> w10
    stop <- "stop 2" stop-if-true
    n108 = node-c288() -> ()  [unwired: 1 in, 1 out]
    n109 = String To IP(1:"255.255.255.255" ("name")) -> (0:w355:u32)
    n110 = UDP Write(address=w355, port or service name=u16 1005, connection ID=w356, data in=w352) -> (3:w350:refnum<k16>)  [unwired: 2 in, 1 out]
    n111 = node-c288() -> ()  [unwired: 1 in, 1 out]
  }
  n112 = Flatten To String(anything=w23, byte order (0:big-endian, network order)=T3."big-endian, network order") -> (data string=w26:string)  [unwired: 2 in, 2 out]
  n113 = Flatten To String(anything=w57, byte order (0:big-endian, network order)=T3."big-endian, network order") -> (data string=w60:string)  [unwired: 2 in, 2 out]
  n114 = Flatten To String(anything=w19, byte order (0:big-endian, network order)=T3."big-endian, network order") -> (data string=w43:string)  [unwired: 2 in, 2 out]
  n115 = Flatten To String(anything=w48, byte order (0:big-endian, network order)=T3."big-endian, network order") -> (data string=w51:string)  [unwired: 2 in, 2 out]
  n116 = Flatten To String(anything=w33, byte order (0:big-endian, network order)=T3."big-endian, network order") -> (data string=w36:string)  [unwired: 2 in, 2 out]
  n117 = Flatten To String(anything=8 ("number"), byte order (0:big-endian, network order)=T3."big-endian, network order") -> (data string=w29:string)  [unwired: 2 in, 2 out]
  n118 = Flatten To String(anything=4 ("number"), byte order (0:big-endian, network order)=T3."big-endian, network order") -> (data string=w63:string)  [unwired: 2 in, 2 out]
  n119 = Flatten To String(anything=6 ("number"), byte order (0:big-endian, network order)=T3."big-endian, network order") -> (data string=w46:string)  [unwired: 2 in, 2 out]
  n120 = Flatten To String(anything=5 ("number"), byte order (0:big-endian, network order)=T3."big-endian, network order") -> (data string=w54:string)  [unwired: 2 in, 2 out]
  n121 = Flatten To String(anything=7 ("number"), byte order (0:big-endian, network order)=T3."big-endian, network order") -> (data string=w39:string)  [unwired: 2 in, 2 out]
  n122 = Concatenate Strings(w29, w26) -> (w27:string)
  n123 = timed-loop {
    tunnel: w6 -> [w365]
    tunnel: w27 -> [w361]
    timing: w88 -> [_]
    timing-out: [_] -> w87
    tunnel: [w359] -> w16
    stop <- "stop 17" stop-if-true
    n124 = node-c288() -> ()  [unwired: 1 in, 1 out]
    n125 = String To IP(1:"255.255.255.255" ("name")) -> (0:w364:u32)
    n126 = UDP Write(address=w364, port or service name=u16 1005, connection ID=w365, data in=w361) -> (3:w359:refnum<k16>)  [unwired: 2 in, 1 out]
    n127 = node-c288() -> ()  [unwired: 1 in, 1 out]
  }
  n128 = Concatenate Strings(w63, w60) -> (w61:string)
  n129 = timed-loop {
    tunnel: w6 -> [w374]
    tunnel: w61 -> [w370]
    timing: w96 -> [_]
    timing-out: [_] -> w95
    tunnel: [w368] -> w12
    stop <- "stop 8" stop-if-true
    n130 = node-c288() -> ()  [unwired: 1 in, 1 out]
    n131 = String To IP(1:"255.255.255.255" ("name")) -> (0:w373:u32)
    n132 = UDP Write(address=w373, port or service name=u16 1005, connection ID=w374, data in=w370) -> (3:w368:refnum<k16>)  [unwired: 2 in, 1 out]
    n133 = node-c288() -> ()  [unwired: 1 in, 1 out]
  }
  n134 = Concatenate Strings(w46, w43) -> (w44:string)
  n135 = timed-loop {
    tunnel: w6 -> [w383]
    tunnel: w44 -> [w379]
    timing: w92 -> [_]
    timing-out: [_] -> w91
    tunnel: [w377] -> w14
    stop <- "stop 13" stop-if-true
    n136 = node-c288() -> ()  [unwired: 1 in, 1 out]
    n137 = String To IP(1:"255.255.255.255" ("name")) -> (0:w382:u32)
    n138 = UDP Write(address=w382, port or service name=u16 1005, connection ID=w383, data in=w379) -> (3:w377:refnum<k16>)  [unwired: 2 in, 1 out]
    n139 = node-c288() -> ()  [unwired: 1 in, 1 out]
  }
  n140 = Concatenate Strings(w54, w51) -> (w52:string)
  n141 = timed-loop {
    tunnel: w6 -> [w392]
    tunnel: w52 -> [w388]
    timing: w94 -> [_]
    timing-out: [_] -> w93
    tunnel: [w386] -> w13
    stop <- "stop 11" stop-if-true
    n142 = node-c288() -> ()  [unwired: 1 in, 1 out]
    n143 = String To IP(1:"255.255.255.255" ("name")) -> (0:w391:u32)
    n144 = UDP Write(address=w391, port or service name=u16 1005, connection ID=w392, data in=w388) -> (3:w386:refnum<k16>)  [unwired: 2 in, 1 out]
    n145 = node-c288() -> ()  [unwired: 1 in, 1 out]
  }
  n146 = Concatenate Strings(w39, w36) -> (w37:string)
  n147 = timed-loop {
    tunnel: w6 -> [w401]
    tunnel: w37 -> [w397]
    timing: w90 -> [_]
    timing-out: [_] -> w89
    tunnel: [w395] -> w15
    stop <- "stop 15" stop-if-true
    n148 = node-c288() -> ()  [unwired: 1 in, 1 out]
    n149 = String To IP(1:"255.255.255.255" ("name")) -> (0:w400:u32)
    n150 = UDP Write(address=w400, port or service name=u16 1005, connection ID=w401, data in=w397) -> (3:w395:refnum<k16>)  [unwired: 2 in, 1 out]
    n151 = node-c288() -> ()  [unwired: 1 in, 1 out]
  }
  n152 = Flatten To String(anything=w21, byte order (0:big-endian, network order)=T3."big-endian, network order") -> (data string=w67:string)  [unwired: 2 in, 2 out]
  n153 = Flatten To String(anything=3 ("number"), byte order (0:big-endian, network order)=T3."big-endian, network order") -> (data string=w70:string)  [unwired: 2 in, 2 out]
  n154 = Concatenate Strings(w70, w67) -> (w68:string)
  n155 = timed-loop {
    tunnel: w6 -> [w410]
    tunnel: w68 -> [w406]
    timing: w98 -> [_]
    timing-out: [_] -> w97
    tunnel: [w404] -> w11
    stop <- "stop 6" stop-if-true
    n156 = node-c288() -> ()  [unwired: 1 in, 1 out]
    n157 = String To IP(1:"255.255.255.255" ("name")) -> (0:w409:u32)
    n158 = UDP Write(address=w409, port or service name=u16 1005, connection ID=w410, data in=w406) -> (3:w404:refnum<k16>)  [unwired: 2 in, 1 out]
    n159 = node-c288() -> ()  [unwired: 1 in, 1 out]
  }
  n160 = node-c288(w97) -> ()  [unwired: 1 out]
  n161 = node-c288(w87) -> ()  [unwired: 1 out]
  n162 = node-c288(w95) -> ()  [unwired: 1 out]
  n163 = node-c288(w101) -> ()  [unwired: 1 out]
  n164 = node-c288(w91) -> ()  [unwired: 1 out]
  n165 = node-c288(w93) -> ()  [unwired: 1 out]
  n166 = node-c288(w89) -> ()  [unwired: 1 out]
  n167 = UDP Close(connection ID=w12) -> ()  [unwired: 1 in, 2 out]
  n168 = UDP Close(connection ID=w11) -> ()  [unwired: 1 in, 2 out]
  n169 = UDP Close(connection ID=w10) -> ()  [unwired: 1 in, 2 out]
  n170 = UDP Close(connection ID=w16) -> ()  [unwired: 1 in, 2 out]
  n171 = UDP Close(connection ID=w14) -> ()  [unwired: 1 in, 2 out]
  n172 = UDP Close(connection ID=w15) -> ()  [unwired: 1 in, 2 out]
  n173 = UDP Close(connection ID=w13) -> ()  [unwired: 1 in, 2 out]
  n174 = node-c288(w99) -> ()  [unwired: 1 out]
  n175 = UDP Close(connection ID=w9) -> ()  [unwired: 1 in, 2 out]
